vi "test_Path (userdoc).vi"(8 "error in (no error)":errorcluster, 11 "TestCase in":refnum<class "Test Read File.lvclass">) -> (0 "error out":errorcluster, 3 "TestCase out":refnum<class "Test Read File.lvclass">)   [LabVIEW 2019, in "Test Read File.lvclass"]
uses:
  Test Read File.lvclass
  C:/Program Files/National Instruments/LabVIEW 2024/vi.lib/Astemes/LUnit/Test Case.lvclass
  <vilib>/Utility/sysdir.llb/System Directory Type.ctl
  Test Read File.lvclass/Test Read File.ctl
  <vilib>/Astemes/LUnit/Test Case.lvclass/Test Case.ctl
  67e7a72a-9ea7-4747-bee2-ed7f34b0ed5b.vi
  <vilib>/Astemes/LUnit/Core/LUnit Test Case/Private/Append Pass Result.vi
  <vilib>/Astemes/LUnit/Core/LUnit Test Case/Private/Append Fail Result.vi
  67e7a72a-9ea7-4747-bee2-ed7f34b0ed5b.vi/9c5d11cd-9439-4240-a1ee-d9baace9c924.vi
  <vilib>/Astemes/LUnit/Core/LUnit Test Case/Private/Run In UI.vi
  <vilib>/Utility/error.llb/Clear Errors.vi
  Read/Read Section - Path.vi
  TSC File IO.lvlib
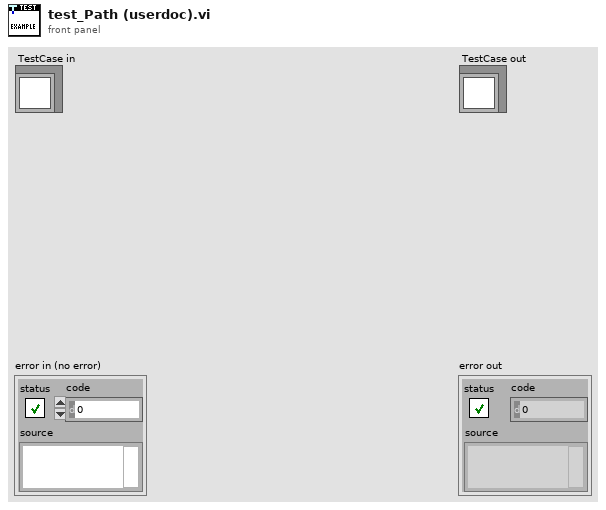
[diagram p1: front panel]
types:
  T1 = typedef "System Directory Type.ctl" = i32
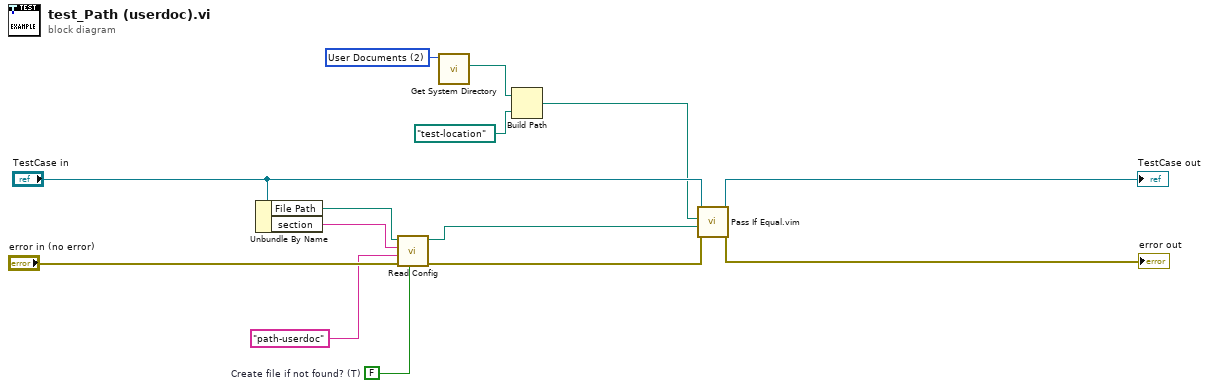
[diagram p0: block diagram]
diagram:
  w5 = T1 2 items=["User Home"=0, "User Desktop"=1, "User Documents"=2, "User Application Data"=3, "User Preferences"=4, "User Temporary"=5, "Public Documents"=6, "Public Application Data"=7, "Public Preferences"=8, "Public Cache"=13, "System Core Libraries"=9, "System Installed Libraries"=10, "Application Files"=11, "Boot Volume Root"=12] ("system directory type")
  w9 = FALSE  # Create file if not found? (T)
  n1 = Unbundle By Name("TestCase in") -> ("File Path"=w1:path, "section"=w2:string)
  n2 = call-poly "Read Config.vi"("Create file if not found? (T)"=w9, "error in (no error)"="error in (no error)", "key"="path-userdoc", "section"=w2, "Path"=w1) -> ("error out"=w8:errorcluster, "value"=w7:path)  [unwired: 5 in]
  n3 = call <vilib>:"Get System Directory.vi"("system directory type"=w5) -> ("system directory"=w4:path)  [unwired: 10 in]
  n4 = Build Path(base path=w4, name or relative path=path "test-location") -> (appended path=w3:path)
  n5 = call "Pass If Equal.vim"("error in (no error)"=w8, "Actual"=w7, "Expected"=w3, "LUnit Test Case In"="TestCase in") -> ("error out"=→"error out":errorcluster, "LUnit Test Case Out"=→"TestCase out":refnum<class "Test Read File.lvclass">)  [unwired: 6 in]
